vi "DB_EscribeTablaTHD.vi"(8 "error in (no error)":errorcluster, 9 "THD_cluster":T1, 10 "Equipo_Medicion":T2={"ID_EQUIPO"=0, "IP_EQUIPO"="", "NOMBRE_EQUIPO"="", "ESTADO_EQUIPO"="", "DESCRIPCION"="", "ID_MEDICION"=0, "ESTADO_MEDICION"="", "TIEMPO_MEDICION"="12-02-2019 18:41"}, 11 "db in":T3) -> (0 "error out":errorcluster, 3 "db out":T3)   [LabVIEW 2018]
uses:
  <vilib>/addons/database/Connection.llb/Conn ObjectReference.ctl
  Controls/Equipos_Medicion_cluster.ctl
  Controls/THD_cluster.ctl
  <vilib>/addons/database/Connection.llb/Conn Execute.vi
  <vilib>/addons/database/Recordset.llb/Rec Destroy - Connection.vi
  <vilib>/addons/database/NI_Database_API.lvlib
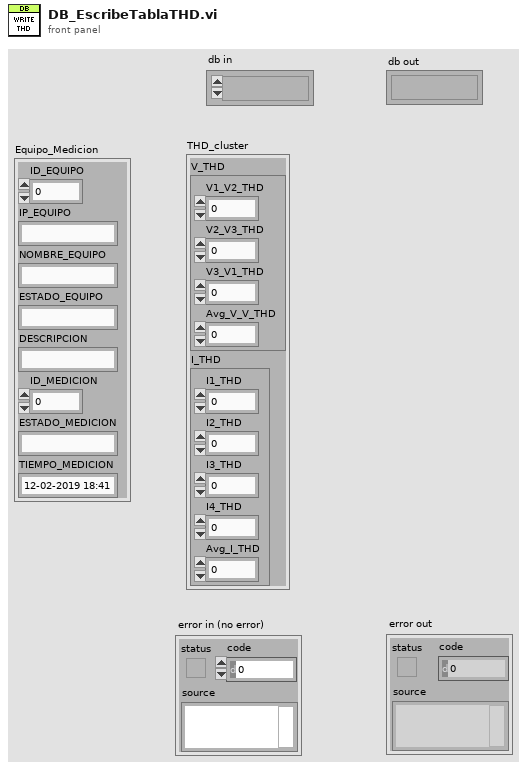
[diagram p1: front panel]
types:
  T1 = typedef "THD_cluster.ctl" = cluster{"V_THD":cluster{"V1_V2_THD":sgl, "V2_V3_THD":sgl, "V3_V1_THD":sgl, "Avg_V_V_THD":sgl}, "I_THD":cluster{"I1_THD":sgl, "I2_THD":sgl, "I3_THD":sgl, "I4_THD":sgl, "Avg_I_THD":sgl}}
  T2 = typedef "Equipos_Medicion_cluster.ctl" = cluster{"ID_EQUIPO":i32, "IP_EQUIPO":string, "NOMBRE_EQUIPO":string, "ESTADO_EQUIPO":string, "DESCRIPCION":string, "ID_MEDICION":i32, "ESTADO_MEDICION":string, "TIEMPO_MEDICION":string}
  T3 = typedef "NI_Database_API.lvlib/Conn ObjectReference.ctl" = refnum<k1>
  T4 = cluster{"V1_V2_THD":sgl, "V2_V3_THD":sgl, "V3_V1_THD":sgl, "Avg_V_V_THD":sgl}
  T5 = cluster{"I1_THD":sgl, "I2_THD":sgl, "I3_THD":sgl, "I4_THD":sgl, "Avg_I_THD":sgl}
  T6 = typedef "NI_Database_API.lvlib/Rec ObjectReference.ctl" = refnum<k1>
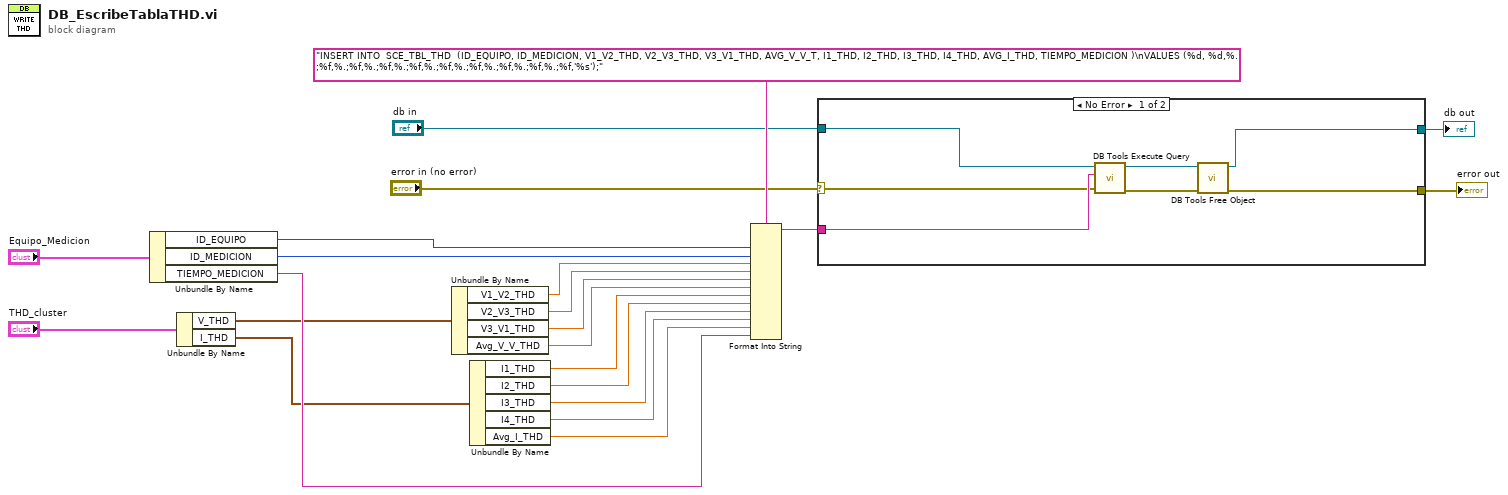
[diagram p0: block diagram]
diagram:
  n1 = Unbundle By Name("Equipo_Medicion") -> ("ID_EQUIPO"=w18:i32, "ID_MEDICION"=w17:i32, "TIEMPO_MEDICION"=w7:string)
  n2 = Unbundle By Name("THD_cluster") -> ("V_THD"=w6:T4, "I_THD"=w5:T5)
  n3 = Unbundle By Name(w6) -> ("V1_V2_THD"=w16:sgl, "V2_V3_THD"=w15:sgl, "V3_V1_THD"=w14:sgl, "Avg_V_V_THD"=w13:sgl)
  n4 = Unbundle By Name(w5) -> ("I1_THD"=w12:sgl, "I2_THD"=w11:sgl, "I3_THD"=w10:sgl, "I4_THD"=w9:sgl, "Avg_I_THD"=w8:sgl)
  n5 = Format Into String(format string="INSERT INTO  SCE_TBL_THD  (ID_EQUIPO, ID_MEDICION, V1_V2_THD, V2_V3_THD, V3_V1_THD, AVG_V_V_T, I1_THD, I2_THD, I3_THD, I4_THD, AVG_I_THD, TIEMPO_MEDICION )\nVALUES (%d, %d,%.;%f,%.;%f,%.;%f,%.;%f,%.;%f,%.;%f,%.;%f,%.;%f,%.;%f,'%s');" ("SQL"), w18, w17, w16, w15, w14, w13, w12, w11, w10, w9, w8, w7) -> (resulting string=w22:string)  [unwired: 2 in, 1 out]
  n6 = case shown="No Error" "error in (no error)" {
    selector: "error in (no error)" -> [w25 w31]
    tunnel: w22 -> [w28 _]
    tunnel: [w27 w31] -> w20
    tunnel: "db in" -> [w24 w30]
    tunnel: [w23 w30] -> w3
    frame No Error {
      n7 = call-poly <vilib>:"DB Tools Execute Query.vi"("error in (no error)"=w25, "SQL query"=w28, "connection reference"=w24) -> ("error out"=w29:errorcluster, "recordset reference"=w26:T6)  [unwired: 5 in]
      n8 = call-poly <vilib>:"DB Tools Free Object.vi"("error in (no error)"=w29, "recordset reference"=w26) -> ("error out"=w27:errorcluster, "connection reference"=w23:T3)  [unwired: 8 in]
    }
    frame Error {
    }
  }
  "error out" <- w20
  "db out" <- w3
